vi "SP Format Value to Fundamental (scalar).vi"(4 "Display Format":T1, 5 "Displayed Value (0)":dbl) -> (1 "Stored Value":dbl)   [LabVIEW 2011]
uses:
  TypeDefs/SP Format.ctl
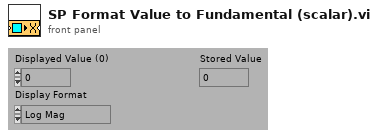
[diagram p1: front panel]
types:
  T1 = typedef "SP Format.ctl" = enum16{"Log Mag", "Lin Mag", "SWR", "Phase", "Expanded Phase", "Delay", "Insertion Loss", "Isolation", "Return Loss"}
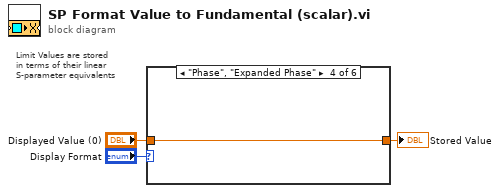
[diagram p0: block diagram]
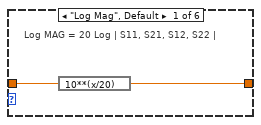
[diagram p2: hidden frame]
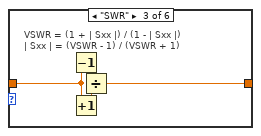
[diagram p4: hidden frame]
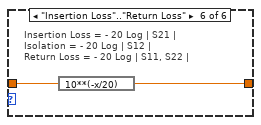
[diagram p6: hidden frame]
diagram:
  # "Limit Values are stored\nin terms of their linear\nS-parameter equivalents"
  n1 = case shown="\"Phase\", \"Expanded Phase\"" "Display Format" {
    tunnel: [w4 w6 w7 w11 w12 w13] -> w1
    tunnel: "Displayed Value (0)" -> [w5 w6 w9 w11 w12 w14]
    frame "Log Mag", Default {
      # "Log MAG = 20 Log | S11, S21, S12, S22 |"
      n2 = expression code="10**(x/20)"(w5) -> (w4:dbl)
    }
    frame "Lin Mag" {
    }
    frame "SWR" {
      # "VSWR = (1 + | Sxx |) / (1 - | Sxx |)\n| Sxx | = (VSWR - 1) / (VSWR + 1)"
      n3 = Decrement(x=w9) -> (x-1=w10:dbl)
      n4 = Increment(x=w9) -> (x+1=w8:dbl)
      n5 = Divide(x=w10, y=w8) -> (x/y=w7:dbl)
    }
    frame "Phase", "Expanded Phase" {
    }
    frame "Delay" {
      # "Group Delay is a derived quantity - we save \nthe number as is..."
    }
    frame "Insertion Loss".."Return Loss" {
      # "Insertion Loss = - 20 Log | S21 |\nIsolation = - 20 Log | S12 |\nReturn Loss = - 20 Log | S11, S22 |"
      n6 = expression code="10**(-x/20)"(w14) -> (w13:dbl)
    }
  }
  "Stored Value" <- w1
